vi "GetCalibrationValues.vi"   [LabVIEW 2019]
uses:
  <vilib>/Rock Robotics/Network Tables/NT Read Boolean.vi
  9c8cb813-da73-458d-a26a-169185133b9c.vi
  9a42c075-bae9-4399-9884-cd741eac9389.vi
  22461746-d047-45df-a0e4-521fa72c0f7c.vi
  <vilib>/Rock Robotics/Network Tables/NT Write Boolean.vi
  DashboardGlobals.vi
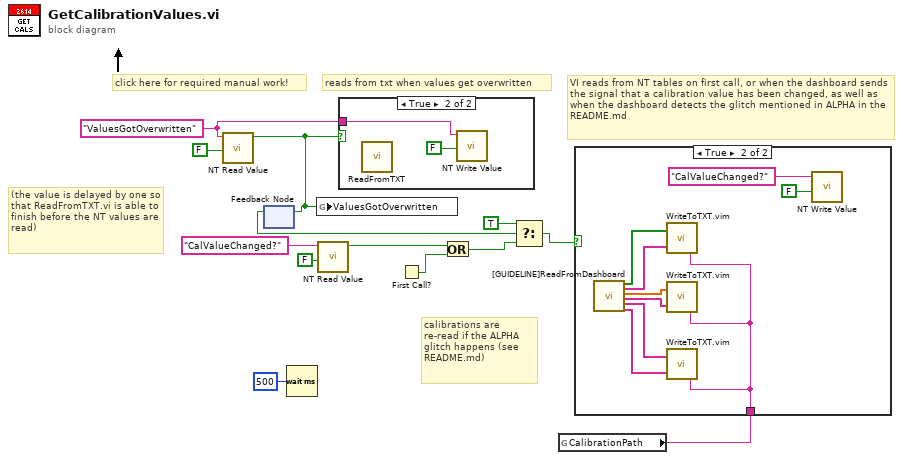
[diagram p0: block diagram]
diagram:
  w1 = "ValuesGotOverwritten" ("Name")
  # "(the value is delayed by one so that ReadFromTXT.vi is able to finish before the NT values are read)"
  # "calibrations are re-read if the ALPHA glitch happens (see README.md)"
  # "reads from txt when values get overwritten"
  # "click here for required manual work!"
  # "VI reads from NT tables on first call, or when the dashboard sends the signal that a calibration value has been changed, as well as when the dashboard detects the glitch mentioned in ALPHA in the README.md"
  n1 = call-poly <vilib>:"NT Read Value.vi"("Default Value"=FALSE, "Name"=w1) -> ("Boolean"=w3:bool)  [unwired: 8 in, 1 out]
  n2 = feedback-in #1(w3) -> ()
  n3 = feedback #1() -> (w2:bool)  [unwired: 1 in]
  n4 = Wait (ms)(milliseconds to wait=u32 500) -> ()  [unwired: 1 out]
  n5 = global write "DashboardGlobals.vi" "ValuesGotOverwritten"(w3) -> ()
  n6 = call-poly <vilib>:"NT Read Value.vi"("Default Value"=FALSE, "Name"="CalValueChanged?") -> ("Boolean"=w11:bool)  [unwired: 8 in, 1 out]
  n7 = case shown="True" w3 {
    tunnel: w1 -> [_ w14]
    frame False {
    }
    frame True {
      n8 = call "ReadFromTXT.vi"() -> ()  [unwired: 12 in]
      n9 = call-poly <vilib>:"NT Write Value.vi"("Boolean"=FALSE ("Default Value"), "Name"=w14) -> ()  [unwired: 9 in, 1 out]
    }
  }
  n10 = First Call?() -> (First Call?: T/F=w8:bool)
  n11 = Or(x=w11, y=w8) -> (x .or. y?=w6:bool)
  n12 = Select(t=TRUE, s=w2, f=w6) -> (s? t:f=w5:bool)
  n13 = global read "DashboardGlobals.vi" "CalibrationPath"() -> (w9:string)
  n14 = case shown="True" w5 {
    tunnel: w9 -> [_ w16]
    frame False {
    }
    frame True {
      n15 = call "[GUIDELINE]ReadFromDashboard.vi"() -> ("boolCalData"=w24:bool[], "boolCalDataNames"=w23:string[], "numCalData"=w22:dbl[], "numCalDataNames"=w21:string[], "stringCalData"=w20:string[], "stringCalDataNames"=w19:string[])  [unwired: 14 in]
      n16 = call "WriteToTXT.vim"("Value Array"=w24, "Name Array"=w23, "path to write to (default /home/lvuser/)"=w16) -> ()  [unwired: 1 in, 1 out]
      n17 = call "WriteToTXT.vim"("Value Array"=w22, "Name Array"=w21, "path to write to (default /home/lvuser/)"=w16) -> ()  [unwired: 1 in, 1 out]
      n18 = call "WriteToTXT.vim"("Value Array"=w20, "Name Array"=w19, "path to write to (default /home/lvuser/)"=w16) -> ()  [unwired: 1 in, 1 out]
      n19 = call-poly <vilib>:"NT Write Value.vi"("Boolean"=FALSE, "Name"="CalValueChanged?") -> ()  [unwired: 9 in, 1 out]
    }
  }
